vi "HexPlot_command.vi"(10 "Dynamic data":T1, 11 "Input parameters":T2={"Measurement type"=enum."Debug", "Sensor type"=enum."HPK_8in_256", "Identifier"="test.txt", "Open after execution?"=FALSE, "Plot after execution?"=FALSE, "Display channel"=0, "Voltage Delay (s)"=0.5, "Switch Delay (s)"=0.01, "VISA resource name source"="", "VISA resource name DMM"="", "VISA resource name LCR"="", "Compliance  Level (A)"=10.0, "Voltage Limit (V)"=1000.0, "Data storage location"="", "Scan voltages"="", "Use source as DMM?"=FALSE, "LCR signal frequenzy (Hz)"=10.0, "DMM device"=enum."Keithley2001", "Sampling number"=1, "Use env. sensors on"=enum."Sensirion sht1x/7x", "Switchboard Handle"=0, "Use Switchboard"=FALSE, "LCR signal voltage (V)"=10000.0, "Repeat"=1, "Scan voltages IV"="", "Scan voltages CV"="", "Hex pad numbers?"=FALSE, "Set measurement type"=enum."Debug", "Custom pad scan"="", "IV voltage Delay (s)"=0.5, "CV voltage Delay (s)"=0.5, "Needle measurement?"=FALSE, "Comments"="test.txt", "LCR signal frequenzy (kHz)"=10.0, "Compliance  Level (uA)"=10.0} {"CV voltage Delay (s)" format="%#_13g"; "IV voltage Delay (s)" format="%#_13g"; "Voltage Limit (V)" format="%#_13g"; "Voltage Delay (s)" format="%#_13g"; "Switch Delay (s)" format="%#_13g"}) -> (0 "HexPlot command":string, 2 "Dynamic data out":T1)   [LabVIEW 2016]
uses:
  Input_parameters.ctl
  Dynamic_data.ctl
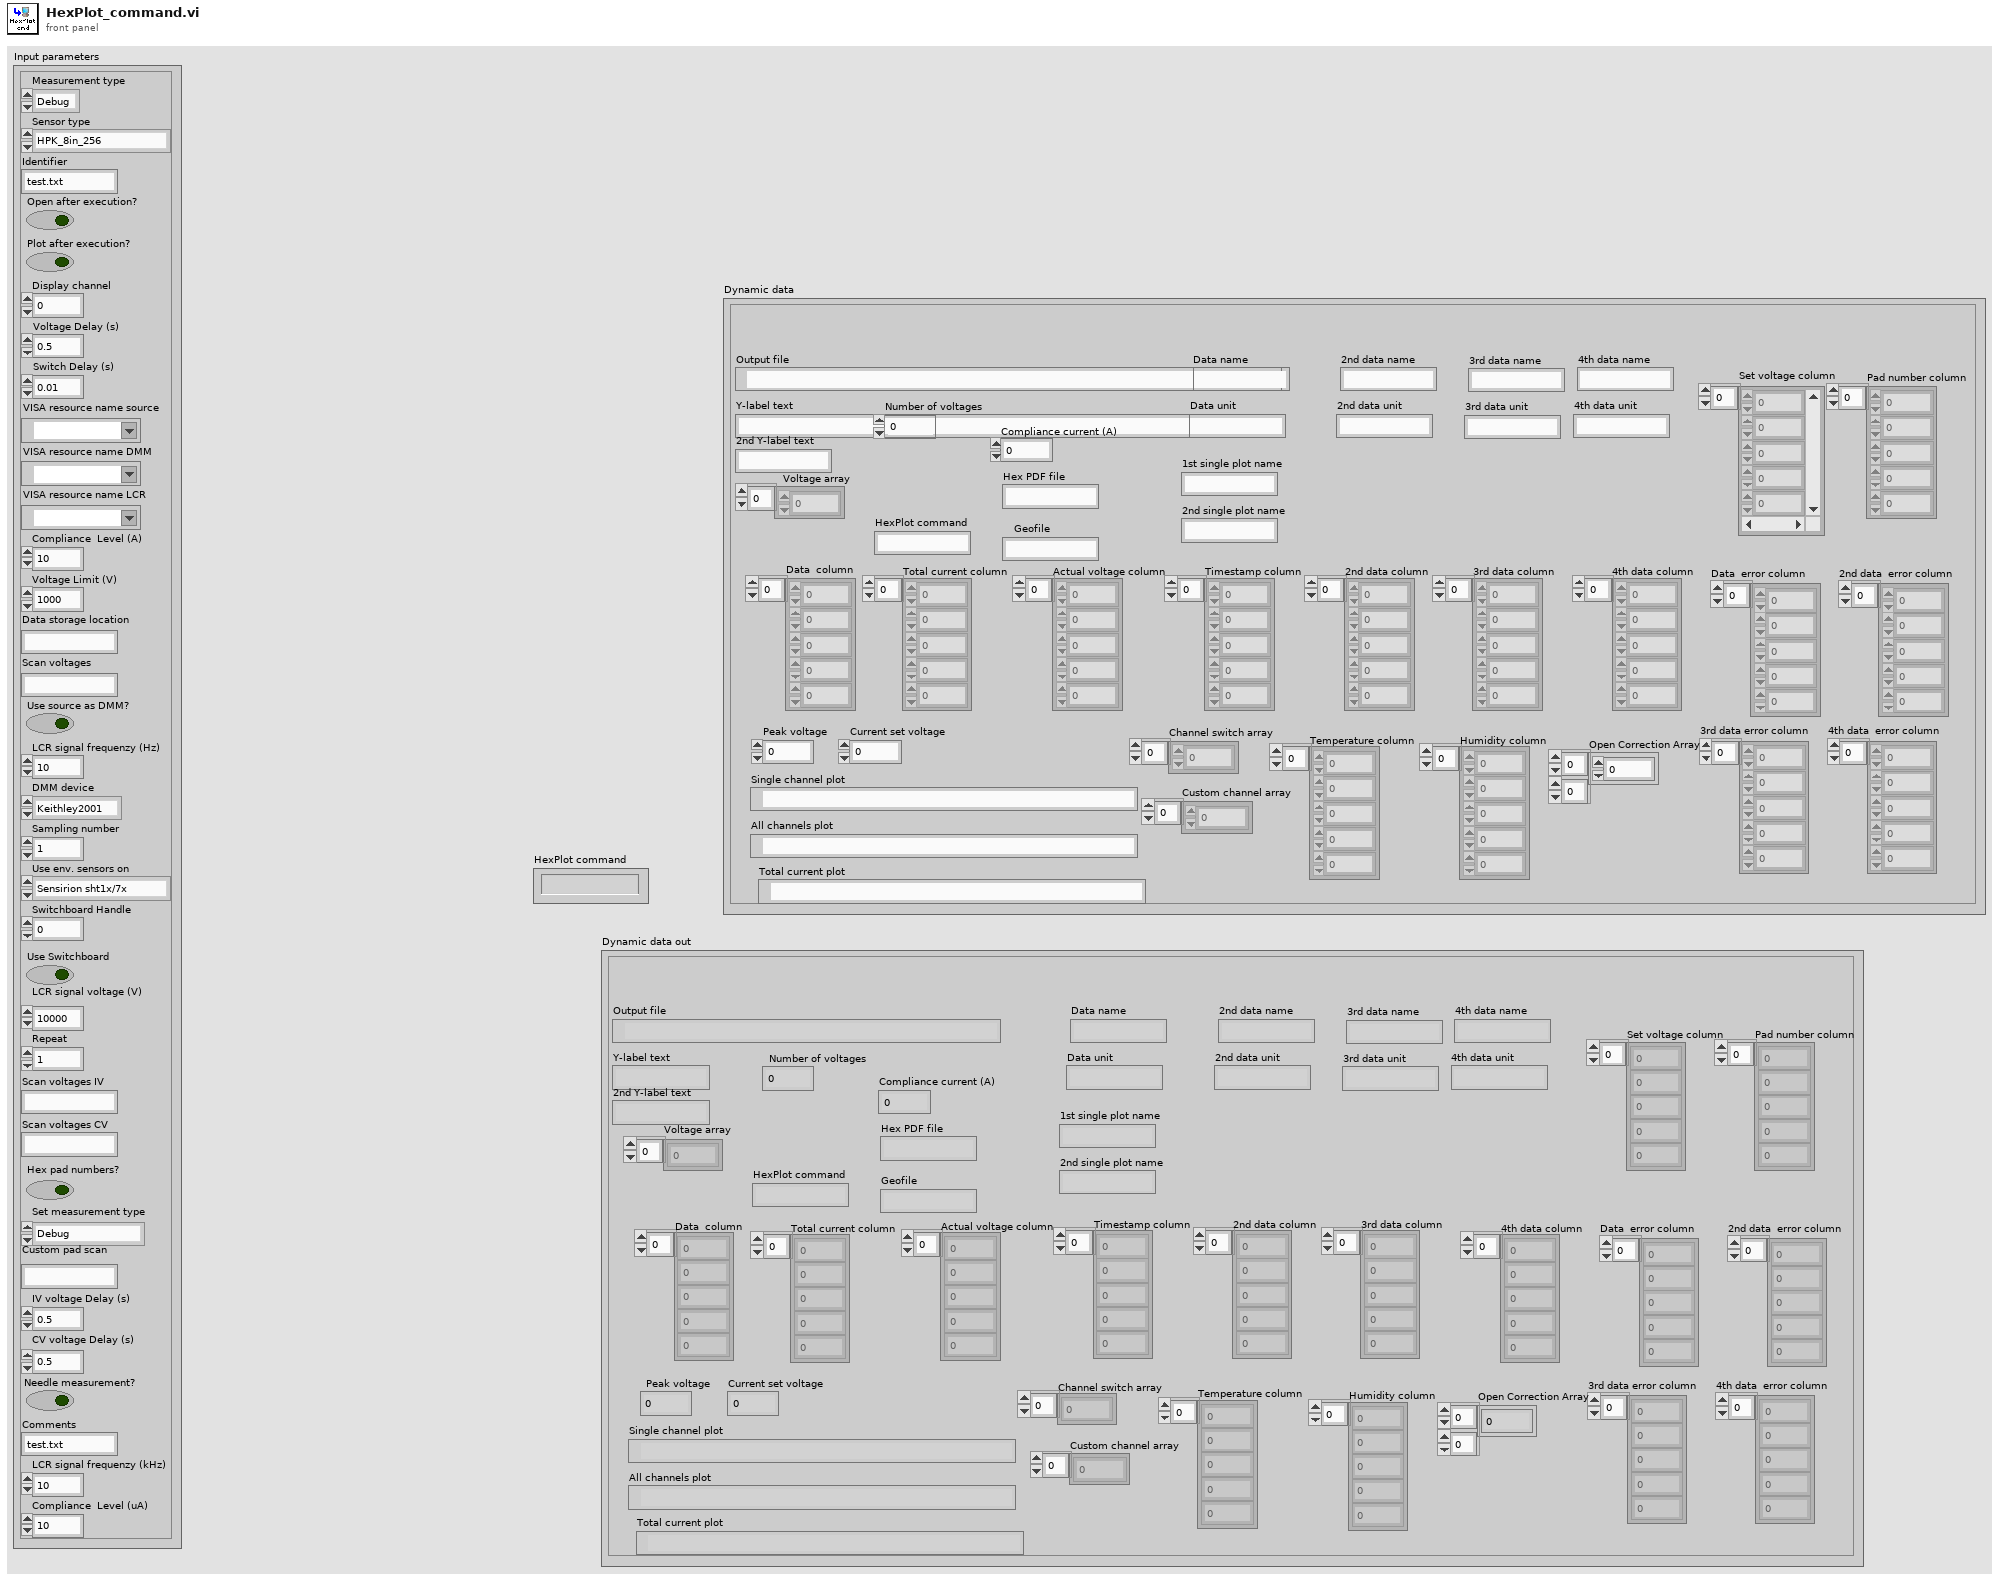
[diagram p1: front panel]
types:
  T1 = typedef "Dynamic_data.ctl" = cluster{"Output file":path, "Y-label text":string, "Current set voltage":dbl, "Set voltage column":dbl[], "Pad number column":dbl[], "Data  column":dbl[], "Number of voltages":i32, "Compliance current (A)":dbl, "Geofile":string, "Peak voltage":dbl, "Hex PDF file":string, "Voltage array":dbl[], "Total current column":dbl[], "Timestamp column":dbl[], "Data name":string, "Data unit":string, "2nd data column":dbl[], "2nd data name":string, "2nd data unit":string, "3rd data column":dbl[], "4th data column":dbl[], "3rd data name":string, "3rd data unit":string, "4th data name":string, "4th data unit":string, "Actual voltage column":dbl[], "2nd Y-label text":string, "Single channel plot":path, "Temperature column":dbl[], "Humidity column":dbl[], "Channel switch array":i32[], "1st single plot name":string, "2nd single plot name":string, "All channels plot":path, "HexPlot command":string, "Custom channel array":i32[], "Data  error column":dbl[], "2nd data  error column":dbl[], "3rd data error column":dbl[], "4th data  error column":dbl[], "Total current plot":path, "Open Correction Array":dbl[][]}
  T2 = typedef "Input_parameters.ctl" = cluster{"Measurement type":enum16{"IV", "CV", "Debug", "Test_contact"}, "Sensor type":enum16{"HPK_6in_135", "HPK_8in_256", "INF_8in_256", "Diode", "HPK_6in_256", "Test capacitances", "Full matrix"}, "Identifier":string, "Open after execution?":bool, "Plot after execution?":bool, "Display channel":i32, "Voltage Delay (s)":dbl, "Switch Delay (s)":dbl, "VISA resource name source":refnum<visa-resource-name>, "VISA resource name DMM":refnum<visa-resource-name>, "VISA resource name LCR":refnum<visa-resource-name>, "Compliance  Level (A)":dbl, "Voltage Limit (V)":dbl, "Data storage location":string, "Scan voltages":string, "Use source as DMM?":bool, "LCR signal frequenzy (Hz)":dbl, "DMM device":enum16{"Keithley2001", "Keithley2450", "Keithley2410", "Keithley6487"}, "Sampling number":i32, "Use env. sensors on":enum16{"Sensirion sht1x/7x", "Switch Matrix", "Probecard"}, "Switchboard Handle":u32, "Use Switchboard":bool, "LCR signal voltage (V)":dbl, "Repeat":i32, "Scan voltages IV":string, "Scan voltages CV":string, "Hex pad numbers?":bool, "Set measurement type":enum16{"IV", "CV", "Debug", "Test_contact", "IV+CV"}, "Custom pad scan":string, "IV voltage Delay (s)":dbl, "CV voltage Delay (s)":dbl, "Needle measurement?":bool, "Comments":string, "LCR signal frequenzy (kHz)":dbl, "Compliance  Level (uA)":dbl}
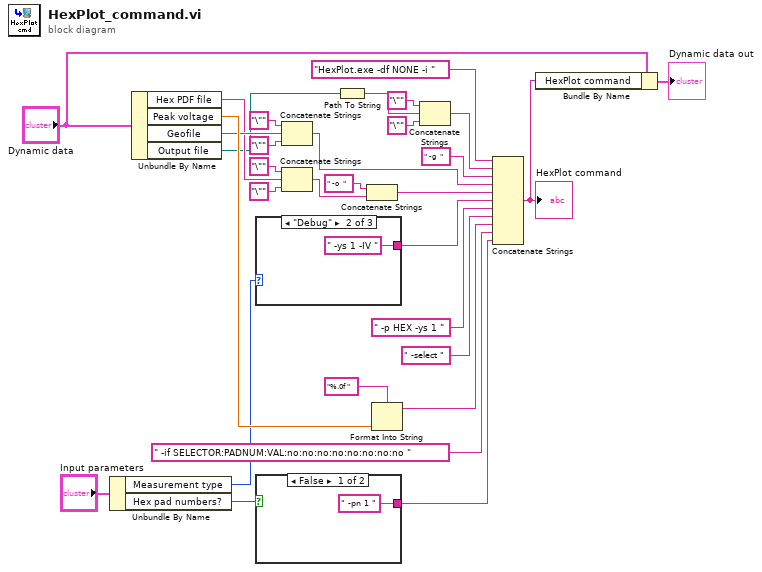
[diagram p0: block diagram]
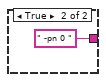
[diagram p2: hidden frame]
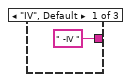
[diagram p3: hidden frame]
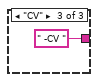
[diagram p4: hidden frame]
diagram:
  n1 = Unbundle By Name("Input parameters") -> ("Measurement type"=w9:enum16{"IV", "CV", "Debug", "Test_contact"}, "Hex pad numbers?"=w6:bool)
  n2 = Unbundle By Name("Dynamic data") -> ("Hex PDF file"=w10:string, "Peak voltage"=w26:dbl, "Geofile"=w14:string, "Output file"=w7:path)
  n3 = case shown="\"Debug\"" w9 {
    tunnel: [" -IV " ("string") " -ys 1 -IV " ("string") " -CV " ("string")] -> w29
    frame "IV", Default {
    }
    frame "Debug" {
    }
    frame "CV" {
    }
  }
  n4 = case shown="False" w6 {
    tunnel: [" -pn 1 " ("string") " -pn 0 " ("string")] -> w5
    frame False {
    }
    frame True {
    }
  }
  n5 = Concatenate Strings("\"" ("string"), w14, "\"" ("string")) -> (w20:string)
  n6 = Concatenate Strings("\"" ("string"), w10, "\"" ("string")) -> (w11:string)
  n7 = Path To String(path=w7) -> (string=w8:string)
  n8 = Concatenate Strings(" -o  " ("string"), w11) -> (w16:string)
  n9 = Format Into String(format string="%.0f ", w26) -> (resulting string=w24:string)  [unwired: 2 in, 1 out]
  n10 = Concatenate Strings("\"" ("string"), w8, "\"" ("string")) -> (w17:string)
  n11 = Concatenate Strings("HexPlot.exe -df NONE -i " ("string"), w17, " -g  " ("string"), w20, w16, w29, " -p HEX -ys 1 " ("string"), " -select " ("string"), w24, " -if SELECTOR:PADNUM:VAL:no:no:no:no:no:no:no:no " ("string"), w5) -> (w1:string)
  "HexPlot command" <- w1
  n12 = Bundle By Name(cluster="Dynamic data", "HexPlot command"=w1) -> (→"Dynamic data out":T1)
